vi "Waveform Flatten.vi"(7 "payload in":u8[](array[numeric]), 8 "error in (no error)":errorcluster, 10 "Data in":T1[](array[typedef]), 11 "CIFFifo in":refnum<class "CIFfifo.lvclass">) -> (0 "error out":errorcluster, 1 "Total Length":i32, 2 "Data out":T1[](array[typedef]), 3 "CIFFifo out":refnum<class "CIFfifo.lvclass">, 5 "payload out":u8[](array[numeric]))   [LabVIEW 2021, in "CIFfifo.lvclass"]
uses:
  CIFfifo.lvclass
  CIFfifo.lvclass/CIFfifo.ctl
  Accessors/Write Payload Length.vi
  Accessors/Read Header.vi
  CIFCore/Common/Utilities/Add Error.vi
  be899675-9489-4ae7-9bdb-bbc908cd9623.vi/c28b0ead-42ad-4072-80a2-aca7f2bd7ce3.vi
  fa4e04b0-1c28-4039-87e0-9391600efeb5.vi/c28b0ead-42ad-4072-80a2-aca7f2bd7ce3.vi
  24dfac9c-4f7b-471b-adb6-3e40fb284e05.vi/c28b0ead-42ad-4072-80a2-aca7f2bd7ce3.vi
  CIFCore/Common/Utilities/Append Error Location.vi
  ChannelCommon.lvlib
  6fdbece9-bad6-4a8e-9bf7-fe1528478dd6.vi
  d5e54e4f-7f1a-40ef-960c-6b2cd585230c.vi
  a071385d-aa0c-48d2-a5ce-3b08816305e6.vi
  typedef/Datatype Waveform.ctl
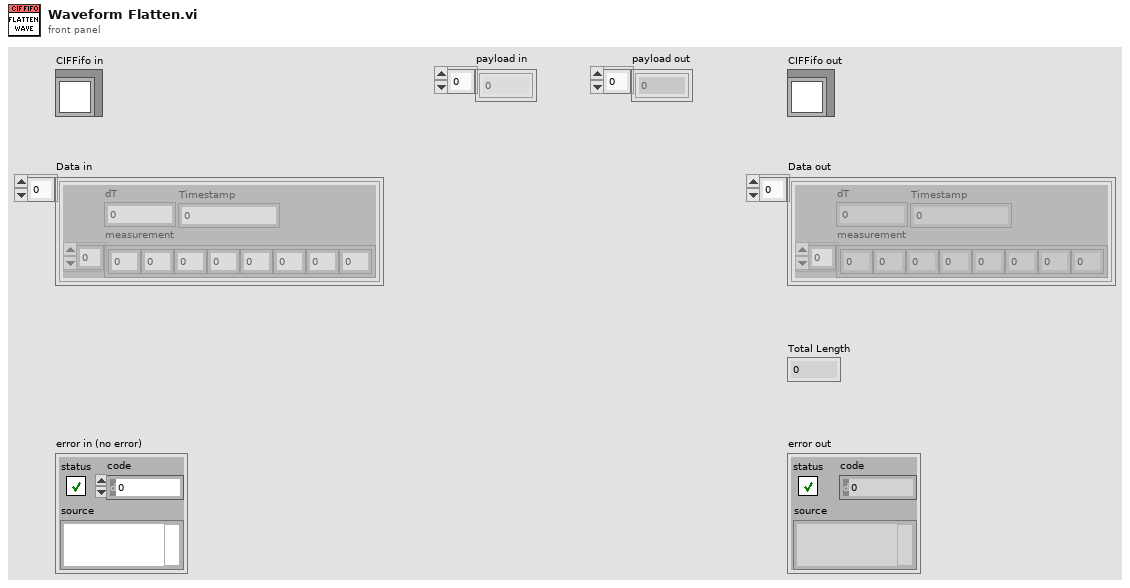
[diagram p1: front panel]
types:
  T1 = typedef "ChannelCommon.lvlib/Datatype Waveform.ctl" = cluster{"measurement":dbl[], "dT":dbl, "Timestamp":u64}
  T2 = typedef "ChannelCommon.lvlib/FIFO Header.ctl" = cluster{"Length":u64, "T0":u64, "T_Out":u64, "T_Tx":u64, "Ctr":u64}
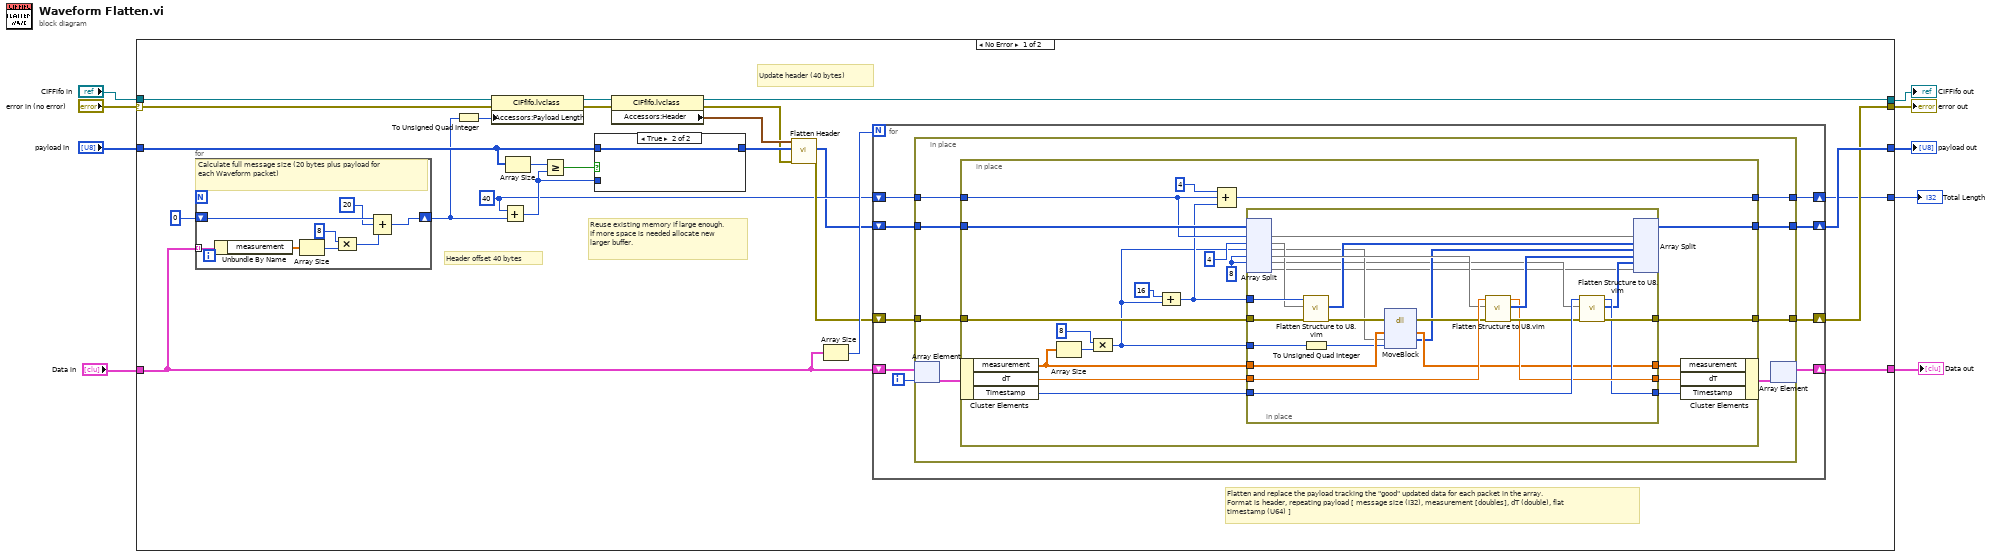
[diagram p0: block diagram]
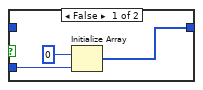
[diagram p2: hidden frame]
diagram:
  n1 = case shown="No Error" "error in (no error)" {
    selector: "error in (no error)" -> [w24 w110]
    tunnel: [w17 w110] -> w8
    tunnel: "Data in" -> [w10 w107]
    tunnel: "CIFFifo in" -> [w33 w109]
    tunnel: [w21 w109] -> w4
    tunnel: [w18 w108] -> w6
    tunnel: "payload in" -> [w25 w108]
    tunnel: [w16 w107] -> w2
    tunnel: [w13 _] -> w1
    frame No Error {
      w15 = 40 ("y")
      # "Flatten and replace the payload tracking the \"good\" updated data for each packet in the array.\nFormat is header, repeating payload [ message size (I32), measurement [doubles], dT (double), flat timestamp (U64) ]"
      # "Header offset 40 bytes"
      # "Update header (40 bytes)"
      # "Reuse existing memory if large enough.  If more space is needed allocate new larger buffer."
      n2 = for {
        tunnel: w10 -> [w41] mode=indexing
        shift-right: [w39] -> w11
        shift-left: 0 -> [w38]
        # "Calculate full message size (20 bytes plus payload for each Waveform packet)"
        n3 = Unbundle By Name(w41) -> ("measurement"=w40:dbl[])
        n4 = Array Size(array=w40) -> (size(s)=w36:i32)
        n5 = Compound Arithmetic op=MULTIPLY(8 ("value"), w36) -> (w35:i32)
        n6 = Compound Arithmetic op=ADD(w38, 20 ("value"), w35) -> (w39:i32)
      }
      n7 = To Unsigned Quad Integer(1:w11) -> (0:w31:u64)
      n8 = property class="CIFfifo.lvclass"(reference=w33, error in=w24, "Accessors:Payload Length"=w31) -> (reference out=w23:refnum<class "CIFfifo.lvclass">, error out=w22:errorcluster)
      n9 = Add(x=w15, y=w11) -> (x+y=w26:i32)
      n10 = Array Size(array=w25) -> (size(s)=w30:i32)
      n11 = Greater Or Equal?(x=w30, y=w26) -> (x >= y?=w29:bool)
      n12 = case shown="True" w29 {
        tunnel: w25 -> [_ w106]
        tunnel: [w103 w106] -> w28
        tunnel: w26 -> [w105 _]
        frame False {
          n13 = Initialize Array(u8 0, w105) -> (w103:u8[])
        }
        frame True {
        }
      }
      n14 = property class="CIFfifo.lvclass"(reference=w23, error in=w22) -> (reference out=w21:refnum<class "CIFfifo.lvclass">, error out=w27:errorcluster, "Accessors:Header"=w32:T2)
      n15 = call "Flatten Header.vi"("error in"=w27, "Flattened Data in"=w28, "Header in"=w32) -> ("error out"=w19:errorcluster, "Flattened Data out"=w14:u8[])  [unwired: 6 in, 1 out]
      n16 = Array Size(array=w10) -> (size(s)=w20:i32)
      n17 = for {
        N: w20 -> [_]
        shift-right: [w50] -> w17
        shift-left: w19 -> [w49]
        shift-right: [w47] -> w18
        shift-left: w14 -> [w48]
        shift-right: [w45] -> w13
        shift-left: w15 -> [w46]
        shift-right: [w42] -> w16
        shift-left: w10 -> [w44]
        i -> [w43]
        n18 = in-place {
          in-place-border: [w58] -> w50
          in-place-border: w49 -> [w57]
          in-place-border: w48 -> [w56]
          in-place-border: [w55] -> w47
          in-place-border: w46 -> [w54]
          in-place-border: [w53] -> w45
          n19 = in-place-array #1(w44, w43) -> (w52:T1)
          n20 = in-place {
            in-place-border: [w78] -> w58
            in-place-border: w57 -> [w77]
            in-place-border: w56 -> [w76]
            in-place-border: [w75] -> w55
            in-place-border: w54 -> [w74]
            in-place-border: [w73] -> w53
            w59 = 8
            n21 = in-place-cluster #2(w52) -> ("measurement"=w68:dbl[], "dT"=w67:dbl, "Timestamp"=w66:u64)
            n22 = Array Size(array=w68) -> (size(s)=w61:i32)
            n23 = Compound Arithmetic op=MULTIPLY(8 ("value"), w61) -> (w60:i32)
            n24 = Compound Arithmetic op=ADD(16 ("value"), w60) -> (w70:i32)
            n25 = Compound Arithmetic op=ADD(4, w74, w70) -> (w73:i32)
            n26 = in-place {
              in-place-border: w66 -> [w99]
              in-place-border: w77 -> [w101]
              in-place-border: [w100] -> w78
              in-place-border: w68 -> [w87]
              in-place-border: w67 -> [w97]
              in-place-border: w70 -> [w94]
              in-place-border: [w86] -> w65
              in-place-border: [w91] -> w64
              in-place-border: [w90] -> w63
              in-place-border: w60 -> [w85]
              n27 = in-place-split #3(w76, w74, 4, w60, w59, w59) -> (w102:u8[], w92:u8[], w83:u8[], w96:u8[], w81:u8[], w79:u8[])
              n28 = call "Flatten Structure to U8.vim"("error in"=w101, "Flattened Data in"=w92, "Data to Flatten in"=w94) -> ("error out"=w89:errorcluster, "Flattened Data out"=w93:u8[])  [unwired: 6 in, 1 out]
              n29 = To Unsigned Quad Integer(1:w85) -> (0:w84:u64)
              n30 = dll-call lib="LabVIEW" fn="MoveBlock"(error in=w89, "source"=w87, "dest"=w83, "size"=w84) -> (error out=w88:errorcluster, "source"=w86:dbl[], "dest"=w82:u8[])  [unwired: 4 in, 1 out]
              n31 = call "Flatten Structure to U8.vim"("error in"=w88, "Flattened Data in"=w96, "Data to Flatten in"=w97) -> ("error out"=w98:errorcluster, "Flattened Data out"=w95:u8[], "Data to Flatten out"=w91:dbl)  [unwired: 6 in]
              n32 = call "Flatten Structure to U8.vim"("error in"=w98, "Flattened Data in"=w81, "Data to Flatten in"=w99) -> ("error out"=w100:errorcluster, "Flattened Data out"=w80:u8[], "Data to Flatten out"=w90:u64)  [unwired: 6 in]
              n33 = in-place-split #3(w102, w93, w82, w95, w80, w79) -> (w75:u8[])  [unwired: 5 out]
            }
            n34 = in-place-cluster #2("measurement"=w65, "dT"=w64, "Timestamp"=w63) -> (w51:T1)
          }
          n35 = in-place-array #1(w51) -> (w42:T1[])  [unwired: 1 out]
        }
      }
    }
    frame Error {
    }
  }
  "error out" <- w8
  "CIFFifo out" <- w4
  "payload out" <- w6
  "Data out" <- w2
  "Total Length" <- w1
